vi "MultiMFC.vi"() -> ()   [LabVIEW 2016]
panel:
  in  "Tab Control":enum32{"Page 1", "Page 2"}(tab)
  in  "Array":cluster{"Setpoint":dbl, "Valve":bool}[](array[cluster]) caption="Nitrogen       Nitrogen       Nitrogen       Nitrogen      Nitrogen         Ethane          Ethane          Ethane\n        100              100               100                30                   5                  0.3                  5                  30" {"Setpoint" min=0.0 max=100.0 step=10.0 scale=0.0..100.0}
  in  "Gas Release Cart":string="GRC-A"
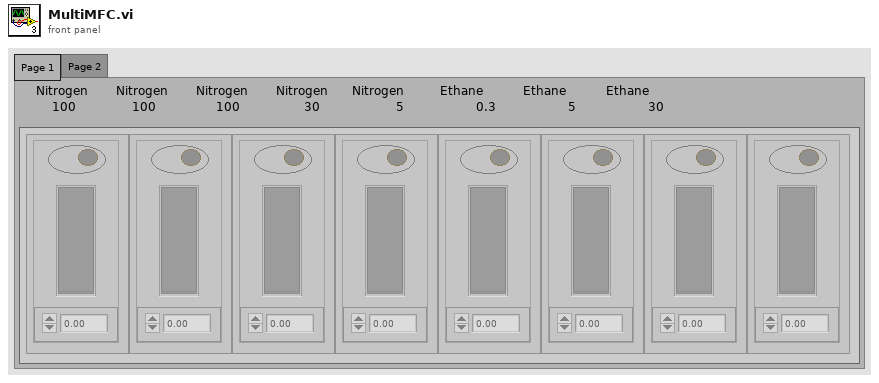
[diagram p1: front panel]
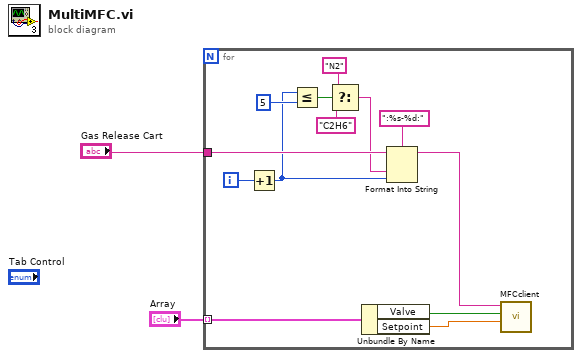
[diagram p0: block diagram]
diagram:
  n1 = for {
    tunnel: "Array" -> [w15] mode=indexing
    tunnel: "Gas Release Cart" -> [w7]
    i -> [w12]
    n2 = Increment(x=w12) -> (x+1=w5:i32)
    n3 = Less Or Equal?(x=w5, y=5) -> (x <= y?=w10:bool)
    n4 = Select(t="N2" ("string"), s=w10, f="C2H6" ("string")) -> (s? t:f=w4:string)
    n5 = Unbundle By Name(w15) -> ("Valve"=w14:bool, "Setpoint"=w13:dbl)
    n6 = Format Into String(format string=":%s-%d:", initial string=w7, w4, w5) -> (resulting string=w3:string)  [unwired: 1 in, 1 out]
    n7 = call "MFCclient.vi"("Setpoint"=w13, "Valve"=w14, "MFCbasename"=w3) -> ()  [unwired: 9 in]
  }
